vi "Actor Core.vi"(8 "error in":errorcluster, 11 "Nested in":refnum<class "Microscope Controller.lvclass">) -> (0 "error out":errorcluster, 3 "Actor out":refnum<class "Actor.lvclass">)   [LabVIEW 2020, in "Microscope.lvlib" / "Microscope Controller.lvlib" / "Microscope Controller.lvclass"]
doc: "(<B>Filename</B>: Actor Framework.lvlib:Actor.lvclass:Actor Core.vi)\n\nReceives messages to the actor, reacts to them, and initiates any error handling that may shut the actor down.\n\nDescendant classes may override this VI to append parallel tasks for the actor to complete while it handles messages. Overrides use the Call Parent Method node."
uses:
  Microscope Controller.lvclass
  C:/Program Files/National Instruments/LabVIEW 2020/vi.lib/ActorFramework/Actor/Actor.lvclass
  <vilib>/ActorFramework/Actor/Actor.lvclass
  <vilib>/ActorFramework/Actor/Actor.lvclass/Actor.ctl
  <vilib>/ActorFramework/Message Enqueuer/Message Enqueuer.lvclass/Message Enqueuer.ctl
  Microscope Controller.lvclass/Microscope Controller.ctl
  <vilib>/ActorFramework/Message Enqueuer/Init from Existing Queue.vi
  <vilib>/ActorFramework/Message Enqueuer/Enqueue.vi
  <vilib>/ActorFramework/Stop Msg/Stop Msg.lvclass
  C:/Program Files/National Instruments/LabVIEW 2020/vi.lib/ActorFramework/Message/Message.lvclass
  Model/HAL Layer/Microscope/Microscope Messages/DebugShowDeviceList Msg/DebugShowDeviceList Msg.lvclass
  <vilib>/ActorFramework/Message Priority Queue/Priority Enqueue.vi
  <vilib>/ActorFramework/Message Enqueuer/Message Enqueuer.lvclass
  E:/Development/DevHardSoftware/MMicroscopyAF/Microscope Controller/Microscope Controller.lvclass
panel:
  in  "Tab Control":T1(tab)
  out "SystemStatus":string
  in  "Full":bool
  in  "Crop":bool
  in  "Scale Bar":bool
  in  "ScaleBarSize":dbl caption="um" min=0.0 max=50.0
  in  "Interval":dbl min=0.0 max=99999.0
  in  "Frames":dbl min=0.0 max=5000.0
  in  "ExposureMs":dbl min=0.0 max=99999.0
  out "AcqTime/min":dbl
  out "DropFrames":dbl
  out "RealFPS":dbl
  out "ImgIndex":dbl
  in  "Save Settings":bool
  in  "Settings":bool
  in  "Snap":bool
  in  "Live":bool
  in  "Acquire":bool
  in  "Stop":bool
  in  "Album":bool
  in  "FrameIndexSroll":i32(c297)
  out "RawImage":T2(plugin-control)
  in  "Exit":bool
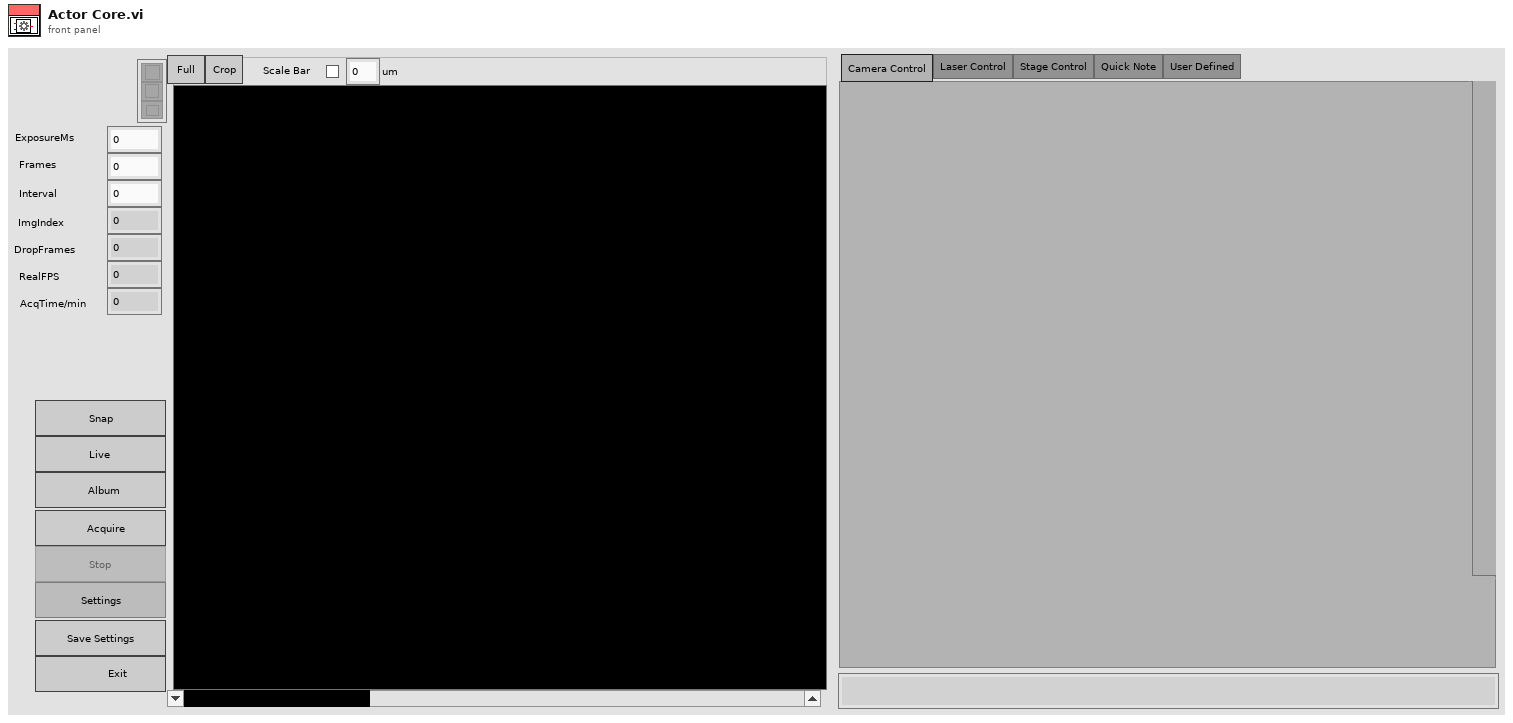
[diagram p1: front panel]
types:
  T1 = enum32{"Camera Control", "Laser Control", "Stage Control", "Quick Note", "User Defined"}
  T2 = typedef "IMAQ Image.ctl" = refnum<image>
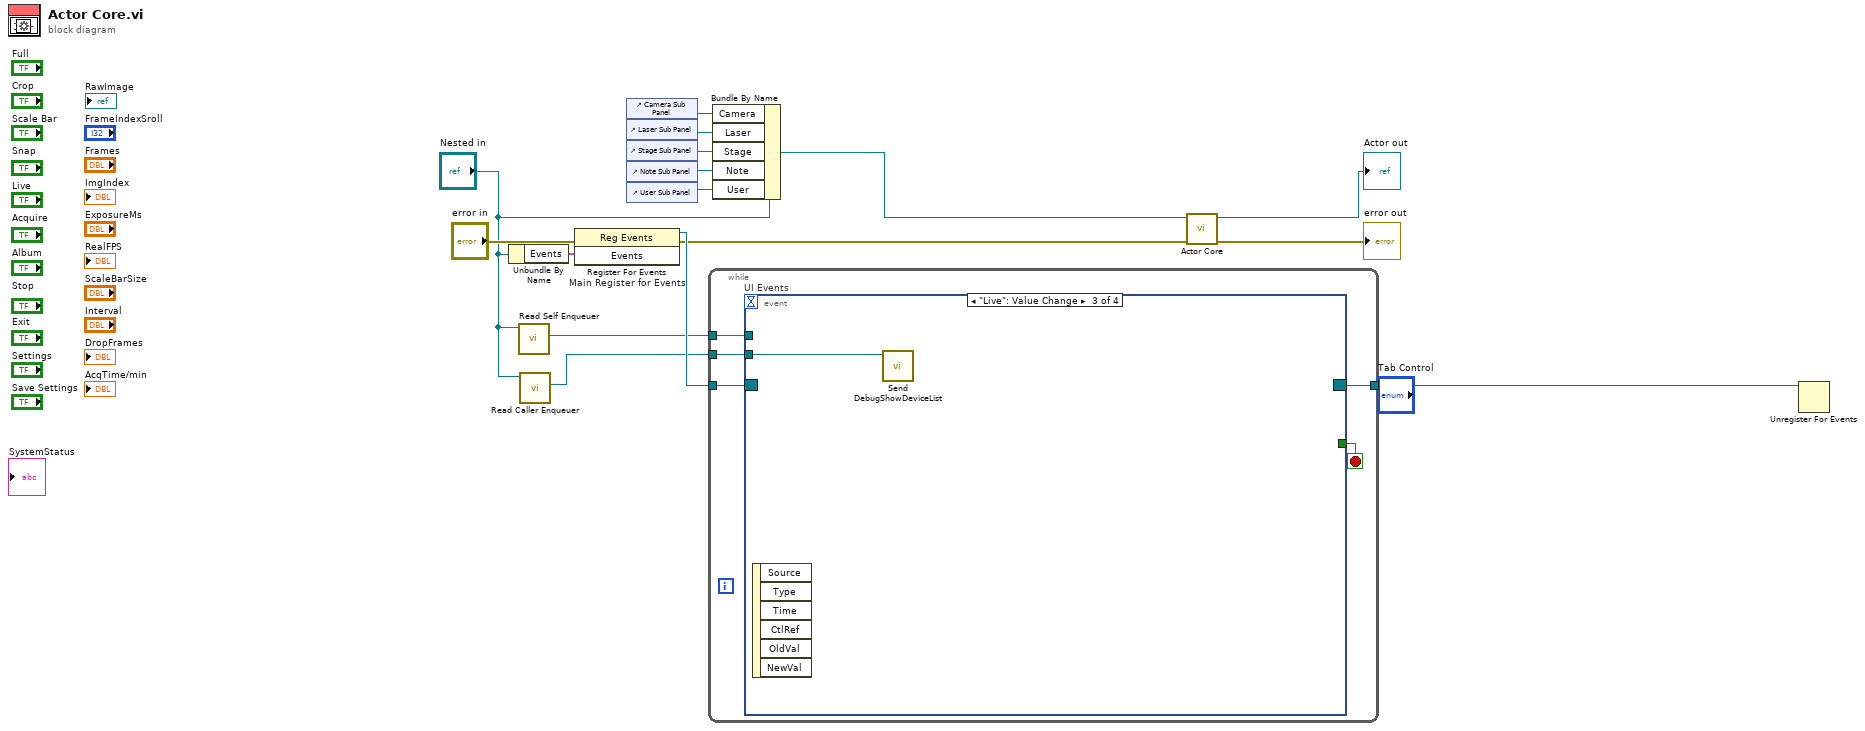
[diagram p0: block diagram]
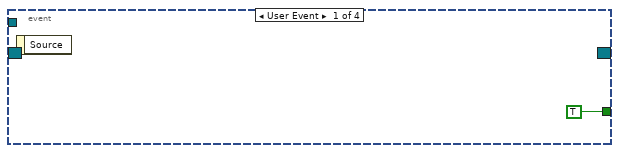
[diagram p2: hidden frame]
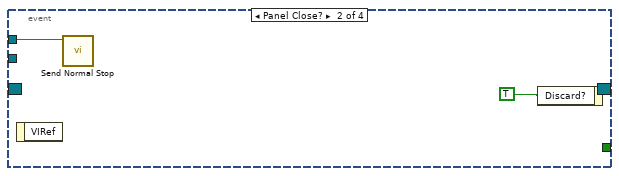
[diagram p3: hidden frame]
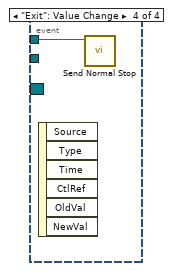
[diagram p4: hidden frame]
diagram:
  n1 = Unbundle By Name("Nested in") -> ("Events"=w13:cluster{"Stop":refnum<user-event>})
  n2 = call <vilib>:"Read Self Enqueuer.vi"("Actor"="Nested in") -> ("Self Enqueuer"=w11:refnum<class "Message Enqueuer.lvclass">)  [unwired: 10 in]
  n3 = call <vilib>:"Read Caller Enqueuer.vi"("Actor"="Nested in") -> ("Caller Enqueuer"=w8:refnum<class "Message Enqueuer.lvclass">)  [unwired: 10 in]
  n4 = register-events "Main Register for Events"(error in="error in", w13) -> (reference out=w14:refnum<event-registration>, error out=w9:errorcluster)  [unwired: 1 in]
  n5 = control-ref of="Camera Sub Panel"() -> (w5:refnum<vi>)
  n6 = control-ref of="Laser Sub Panel"() -> (w4:refnum<vi>)
  n7 = control-ref of="Stage Sub Panel"() -> (w3:refnum<vi>)
  n8 = control-ref of="Note Sub Panel"() -> (w2:refnum<vi>)
  n9 = control-ref of="User Sub Panel"() -> (w1:refnum<vi>)
  n10 = while {
    tunnel: w14 -> [w21]
    tunnel: [w19] -> w12
    tunnel: w11 -> [w18]
    tunnel: w8 -> [w17]
    stop <- w20 stop-if-true
    n11 = event "UI Events" shown="[2] \"Live\": Value Change" {
      selector: w21 -> [_ _ _ _]
      dyn-events: [_ _ _ _] -> w19
      timeout: _ -> [_ _ _ _]
      tunnel: [TRUE _ _ _] -> w20
      tunnel: w18 -> [_ w23 _ w26]
      tunnel: w17 -> [_ _ w25 _]
      event User Event {
        n12 = event-data() -> ()  [unwired: 1 in, 1 out]
      }
      event Panel Close? {
        n13 = event-data() -> ()  [unwired: 1 in, 1 out]
        n14 = call <vilib>:"Send Normal Stop.vi"("Message Enqueuer"=w23) -> ()  [unwired: 10 in, 1 out]
        n15 = event-data("Discard?"=TRUE) -> ()  [unwired: 1 in, 1 out]
      }
      event "Live": Value Change {
        n16 = event-data() -> ()  [unwired: 1 in, 6 out]
        n17 = call "Send DebugShowDeviceList.vi"("Message Enqueuer"=w25) -> ()  [unwired: 9 in, 2 out]
      }
      event "Exit": Value Change {
        n18 = event-data() -> ()  [unwired: 1 in, 6 out]
        n19 = call <vilib>:"Send Normal Stop.vi"("Message Enqueuer"=w26) -> ()  [unwired: 10 in, 1 out]
      }
    }
  }
  n20 = Bundle By Name(cluster="Nested in", "Camera"=w5, "Laser"=w4, "Stage"=w3, "Note"=w2, "User"=w1) -> (w6:refnum<class "Microscope Controller.lvclass">)
  n21 = call-parent "Actor Core.vi"("error in"=w9, "Actor in"=w6) -> ("error out"=→"error out":errorcluster, "Actor out"=→"Actor out":refnum<class "Actor.lvclass">)  [unwired: 8 in]
  n22 = Unregister For Events(event registration refnum=w12) -> ()  [unwired: 1 in, 1 out]
